vi "AgitatorSystem.vi"() -> ()   [LabVIEW 2025]
panel:
  out "AgitatorSystem/AgitatorRPM":dbl caption="Speed  RPM" format="%12.1f"
  out "AgitatorSystem/AgitatorOutput":dbl caption="Motor Dmd" format="%11.2f"
  out "AgitatorSystem/AgitatorState":bool caption="Agitator On"
  # "AGITATOR"
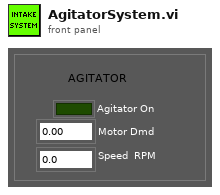
[diagram p1: front panel]
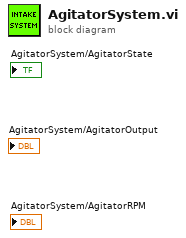
[diagram p0: block diagram]
diagram:
